vi "Display Tree Item.vi"(8 "error in (no error)":errorcluster, 10 "Tag":string, 11 "Application Data in":T1) -> (0 "error out":errorcluster, 3 "Application Data out":T1)   [LabVIEW 2017, in "DSF Configuration Utility.lvlib"]
uses:
  DSF Configuration Utility.lvlib
  Application Data.ctl
  DSF Configuration API/1.0.0/Public/Controls/DSF Config Data RefNum.ctl
  View Mode.ctl
  DSF Configuration API/1.0.0/Public/Read Item/Read Plugin.vi
  DSF Configuration API/1.0.0/Public/Read Item/Read Settings.vi
  DSF Configuration API/1.0.0/Public/Read Item/Read Channel.vi
  DSF Configuration API/1.0.0/Public/Read Item/Read Transfer.vi
  DSF Configuration API/1.0.0/Public/Read Item/Read Group.vi
  DSF Configuration API/1.0.0/DSF Configuration API.lvlib
panel:
  # "App\nData"
  # "App\nData"
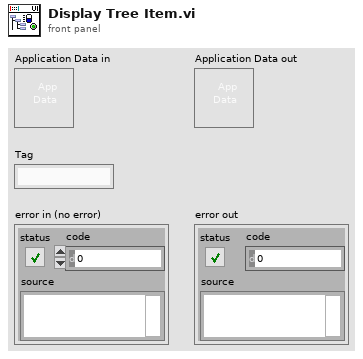
[diagram p1: front panel]
types:
  T1 = typedef "DSF Configuration Utility.lvlib/Application Data.ctl" = cluster{"Item Tree Control":refnum<vi>, "Value Tree Control":refnum<vi>, "DSF Refnum":T2, "Top-Level VI":refnum<vi>, "View State":T3, "menu reference":refnum<k9>}
  T2 = typedef "DSF Configuration API.lvlib/DSF Config Data RefNum.ctl" = refnum<k1>
  T3 = typedef "DSF Configuration Utility.lvlib/View Mode.ctl" = enum16{"Tree", "List"}
  T4 = typedef "DSF Configuration API.lvlib/Version Info.ctl" = cluster{"major":u32, "minor":u32, "fix":u32, "build":string}
  T5 = typedef "DSF Configuration Utility.lvlib/Tree Item Type.ctl" = enum16{"Plugin", "Group", "Transfer", "Channel", "Setting"}
  T6 = typedef "DSF Configuration API.lvlib/DSF Group Info.ctl" = cluster{"direction":i32, "timing":T7, "transfer ids":string[], "settings id":string}
  T7 = typedef "DSF Configuration API.lvlib/DSF Timing Info.ctl" = cluster{"priority":i32, "decimation":i32, "offset":i32}
  T8 = typedef "DSF Configuration API.lvlib/DSF Transfer Info.ctl" = cluster{"byte order":i32, "channel ids":string[], "settings id":string}
  T9 = typedef "DSF Configuration API.lvlib/DSF Channel Info.ctl" = cluster{"count":i32, "offset":i32, "data type":i32, "resource path":string, "settings id":string}
  T10 = typedef "DSF Configuration API.lvlib/DSF Settings Info.ctl" = cluster{"key":string, "value":string}[]
  T11 = typedef "DSF Configuration API.lvlib/DSF Plugin Info.ctl" = cluster{"type":string, "timing":T7, "group ids":string[], "settings id":string}
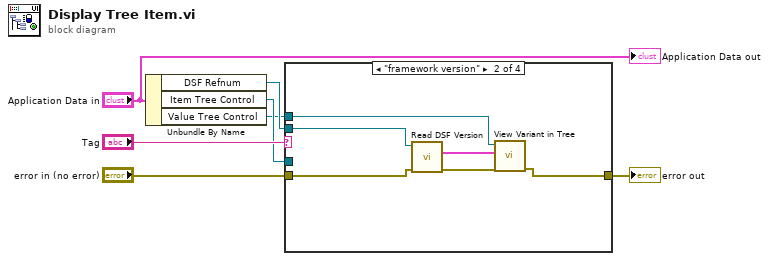
[diagram p0: block diagram]
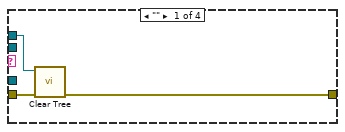
[diagram p2: hidden frame]
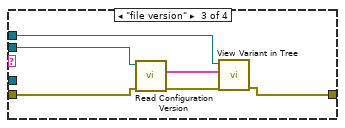
[diagram p3: hidden frame]
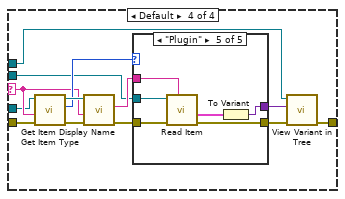
[diagram p4: hidden frame]
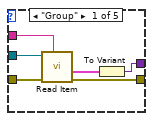
[diagram p5: hidden frame]
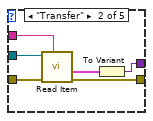
[diagram p6: hidden frame]
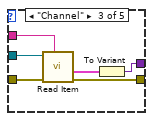
[diagram p7: hidden frame]
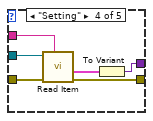
[diagram p8: hidden frame]
diagram:
  n1 = Unbundle By Name("Application Data in") -> ("DSF Refnum"=w5:T2, "Item Tree Control"=w4:refnum<vi>, "Value Tree Control"=w2:refnum<vi>)
  n2 = case shown="\"framework version\"" "Tag" {
    selector: "Tag" -> [_ _ _ w30]
    tunnel: w5 -> [_ w16 w22 w29]
    tunnel: w4 -> [_ _ _ w28]
    tunnel: "error in (no error)" -> [w10 w15 w21 w27]
    tunnel: w2 -> [w8 w11 w17 w24]
    tunnel: [w9 w13 w19 w23] -> w1
    frame "" {
      n3 = call "Clear Tree.vi"("error in (no error)"=w10, "TreeControl in"=w8) -> ("error out"=w9:errorcluster)  [unwired: 9 in]
    }
    frame "framework version" {
      n4 = call "Read DSF Version.vi"("error in (no error)"=w15, "refnum"=w16) -> ("error out"=w14:errorcluster, "dsfversion"=w12:T4)  [unwired: 7 in, 1 out]
      n5 = call "View Variant in Tree.vi"("error in (no error)"=w14, "Variant"=w12, "TreeControl in"=w11) -> ("error out"=w13:errorcluster)  [unwired: 8 in]
    }
    frame "file version" {
      n6 = call "Read Configuration Version.vi"("error in (no error)"=w21, "refnum"=w22) -> ("error out"=w20:errorcluster, "version"=w18:T4)  [unwired: 7 in, 1 out]
      n7 = call "View Variant in Tree.vi"("error in (no error)"=w20, "Variant"=w18, "TreeControl in"=w17) -> ("error out"=w19:errorcluster)  [unwired: 8 in]
    }
    frame Default {
      n8 = call "Get Item Type.vi"("error in (no error)"=w27, "Tag"=w30, "TreeControl in"=w28) -> ("error out"=w34:errorcluster, "Item Type"=w32:T5, "TreeControl out"=w33:refnum<vi>)  [unwired: 6 in]
      n9 = call "Get Item Display Name.vi"("error in (no error)"=w34, "Tag"=w30, "TreeControl in"=w33) -> ("error out"=w35:errorcluster, "display name"=w31:string)  [unwired: 6 in, 1 out]
      n10 = case shown="\"Plugin\"" w32 {
        tunnel: w31 -> [w41 w47 w53 w59 w65]
        tunnel: [w39 w44 w50 w57 w63] -> w26
        tunnel: w35 -> [w38 w45 w51 w58 w64]
        tunnel: w29 -> [w37 w43 w49 w56 w62]
        tunnel: [w36 w42 w48 w54 w61] -> w25
        frame "Group" {
          n11 = call-poly "Read Item.vi"("name"=w41, "error in (no error)"=w38, "refnum"=w37) -> ("error out"=w39:errorcluster, "value"=w40:T6)  [unwired: 5 in, 2 out]
          n12 = To Variant(anything=w40) -> (Variant=w36:variant)
        }
        frame "Transfer" {
          n13 = call-poly "Read Item.vi"("name"=w47, "error in (no error)"=w45, "refnum"=w43) -> ("error out"=w44:errorcluster, "value"=w46:T8)  [unwired: 5 in, 2 out]
          n14 = To Variant(anything=w46) -> (Variant=w42:variant)
        }
        frame "Channel" {
          n15 = call-poly "Read Item.vi"("name"=w53, "error in (no error)"=w51, "refnum"=w49) -> ("error out"=w50:errorcluster, "value"=w52:T9)  [unwired: 5 in, 2 out]
          n16 = To Variant(anything=w52) -> (Variant=w48:variant)
        }
        frame "Setting" {
          n17 = call-poly "Read Item.vi"("name"=w59, "error in (no error)"=w58, "refnum"=w56) -> ("error out"=w57:errorcluster, "value"=w55:T10)  [unwired: 5 in, 2 out]
          n18 = To Variant(anything=w55) -> (Variant=w54:variant)
        }
        frame "Plugin" {
          n19 = call-poly "Read Item.vi"("name"=w65, "error in (no error)"=w64, "refnum"=w62) -> ("error out"=w63:errorcluster, "value"=w60:T11)  [unwired: 5 in, 2 out]
          n20 = To Variant(anything=w60) -> (Variant=w61:variant)
        }
      }
      n21 = call "View Variant in Tree.vi"("error in (no error)"=w26, "Variant"=w25, "TreeControl in"=w24) -> ("error out"=w23:errorcluster)  [unwired: 8 in]
    }
  }
  "error out" <- w1
  "Application Data out" <- "Application Data in"
